vi "Generate and Broadcast Event.vi"(8 "error in (no error)":errorcluster, 10 "Event Data":refnum<class "Event.lvclass">, 11 "View Actor in":refnum<class "View Actor.lvclass">) -> (0 "error out":errorcluster, 3 "View Actor out":refnum<class "View Actor.lvclass">)   [LabVIEW 2017, in "Event Actors.lvlib" / "View Actor.lvclass"]
uses:
  View Actor.lvclass
  C:/Program Files (x86)/National Instruments/LabVIEW 2017/vi.lib/ActorFramework/Actor/Actor.lvclass
  Event/Event.lvclass
  View Actor.lvclass/View Actor.ctl
  <vilib>/ActorFramework/Actor/Actor.lvclass/Actor.ctl
  <vilib>/ActorFramework/Message Enqueuer/Message Enqueuer.lvclass/Message Enqueuer.ctl
  properties/Read Controller Actor Enqueuer.vi
  properties/Read Paused.vi
  properties/Read Receive Only.vi
  <vilib>/ActorFramework/Message Enqueuer/Init from Existing Queue.vi
  <vilib>/ActorFramework/Message Enqueuer/Message Enqueuer.lvclass
  Controller Actor Messages/Handle and Broadcast Event Msg/Handle and Broadcast Event Msg.lvclass
  <vilib>/ActorFramework/Actor/Actor.lvclass
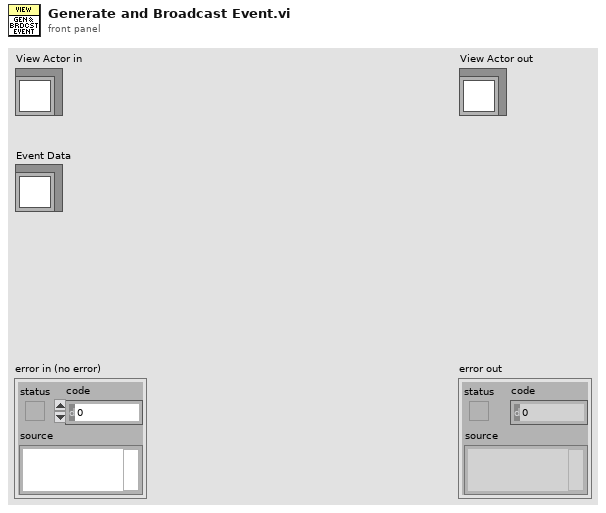
[diagram p1: front panel]
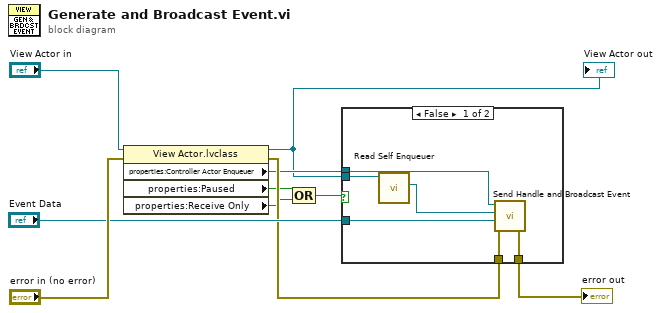
[diagram p0: block diagram]
diagram:
  n1 = property class="View Actor.lvclass"(reference="View Actor in", error in="error in (no error)") -> (reference out=w4:refnum<class "View Actor.lvclass">, error out=w7:errorcluster, "properties:Controller Actor Enqueuer"=w5:refnum<class "Message Enqueuer.lvclass">, "properties:Paused"=w3:bool, "properties:Receive Only"=w2:bool)
  "View Actor out" <- w4
  n2 = Compound Arithmetic op=OR(w3, w2) -> (w1:bool)
  n3 = case shown="False" w1 {
    tunnel: "Event Data" -> [w15 _]
    tunnel: w7 -> [w14 w17]
    tunnel: [w13 w17] -> w6
    tunnel: w5 -> [w12 _]
    tunnel: w4 -> [w11 _]
    frame False {
      n4 = call <vilib>:"Read Self Enqueuer.vi"("Actor"=w11) -> ("Self Enqueuer"=w16:refnum<class "Message Enqueuer.lvclass">)  [unwired: 10 in]
      n5 = call "Send Handle and Broadcast Event.vi"("error in (no error)"=w14, "Event Data"=w15, "View Enqueuer"=w16, "Message Enqueuer in"=w12) -> ("error out"=w13:errorcluster)  [unwired: 6 in, 1 out]
    }
    frame True {
    }
  }
  "error out" <- w6
